vi "WebCam.Connect.vi"(0 "Handle":i32, 11 "ErrorIn":errorcluster) -> (4 "HandleOut":i32, 15 "ErrorOut":errorcluster)   [LabVIEW 2021]
uses:
  User32.WebCam_WM_Events.ctl
  User32.SendMessageA_num.vi
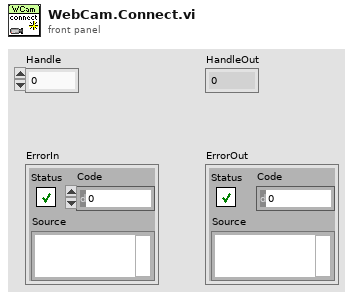
[diagram p1: front panel]
types:
  T1 = typedef "User32.WebCam_WM_Events.ctl" = i32
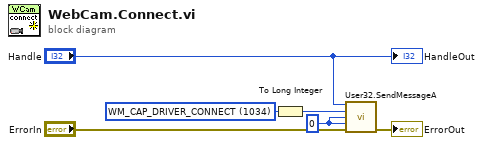
[diagram p0: block diagram]
diagram:
  w3 = T1 1034 items=["WM_CAP_DRIVER_CONNECT"=1034, "WM_CAP_EDIT_COPY"=1054, "WM_CAP_SET_PREVIEW"=1074, "WM_CAP_SET_OVERLAY"=1075, "WM_CAP_SET_PREVIEWRATE"=1076, "WM_CAP_DRIVER_DISCONNECT"=1035, "WM_CAP_SET_SCALE"=1077, "WM_CAP_FILE_SAVEDIB"=1049] ("Ring")
  w1 = 0
  n1 = To Long Integer(number=w3) -> (32bit integer=w2:T1)
  n2 = call-poly "User32.SendMessageA.vi"("HWnd"="Handle", "Msg"=w2, "WParam"=w1, "LParam"=w1, "ErrorIn"="ErrorIn") -> ("ErrorOut"=→"ErrorOut":errorcluster)  [unwired: 9 in, 1 out]
  "HandleOut" <- "Handle"
